vi "Main.vi"() -> ()   [LabVIEW 2019]
uses:
  VIs/Telas.ctl
  VIs/TelaConfig/Configuracao.Variaveis.vi
  Users/Nicole/Downloads/a/ims-desktop/Variaveis/CodOrder.vi
  Users/Nicole/Downloads/a/ims-desktop/Variaveis/WindowAppearance.vi
  Users/Nicole/Downloads/a/ims-desktop/Variaveis/User.vi
panel:
  out "NextScreen":T1
  out "Resize":bool
  out "Code":string
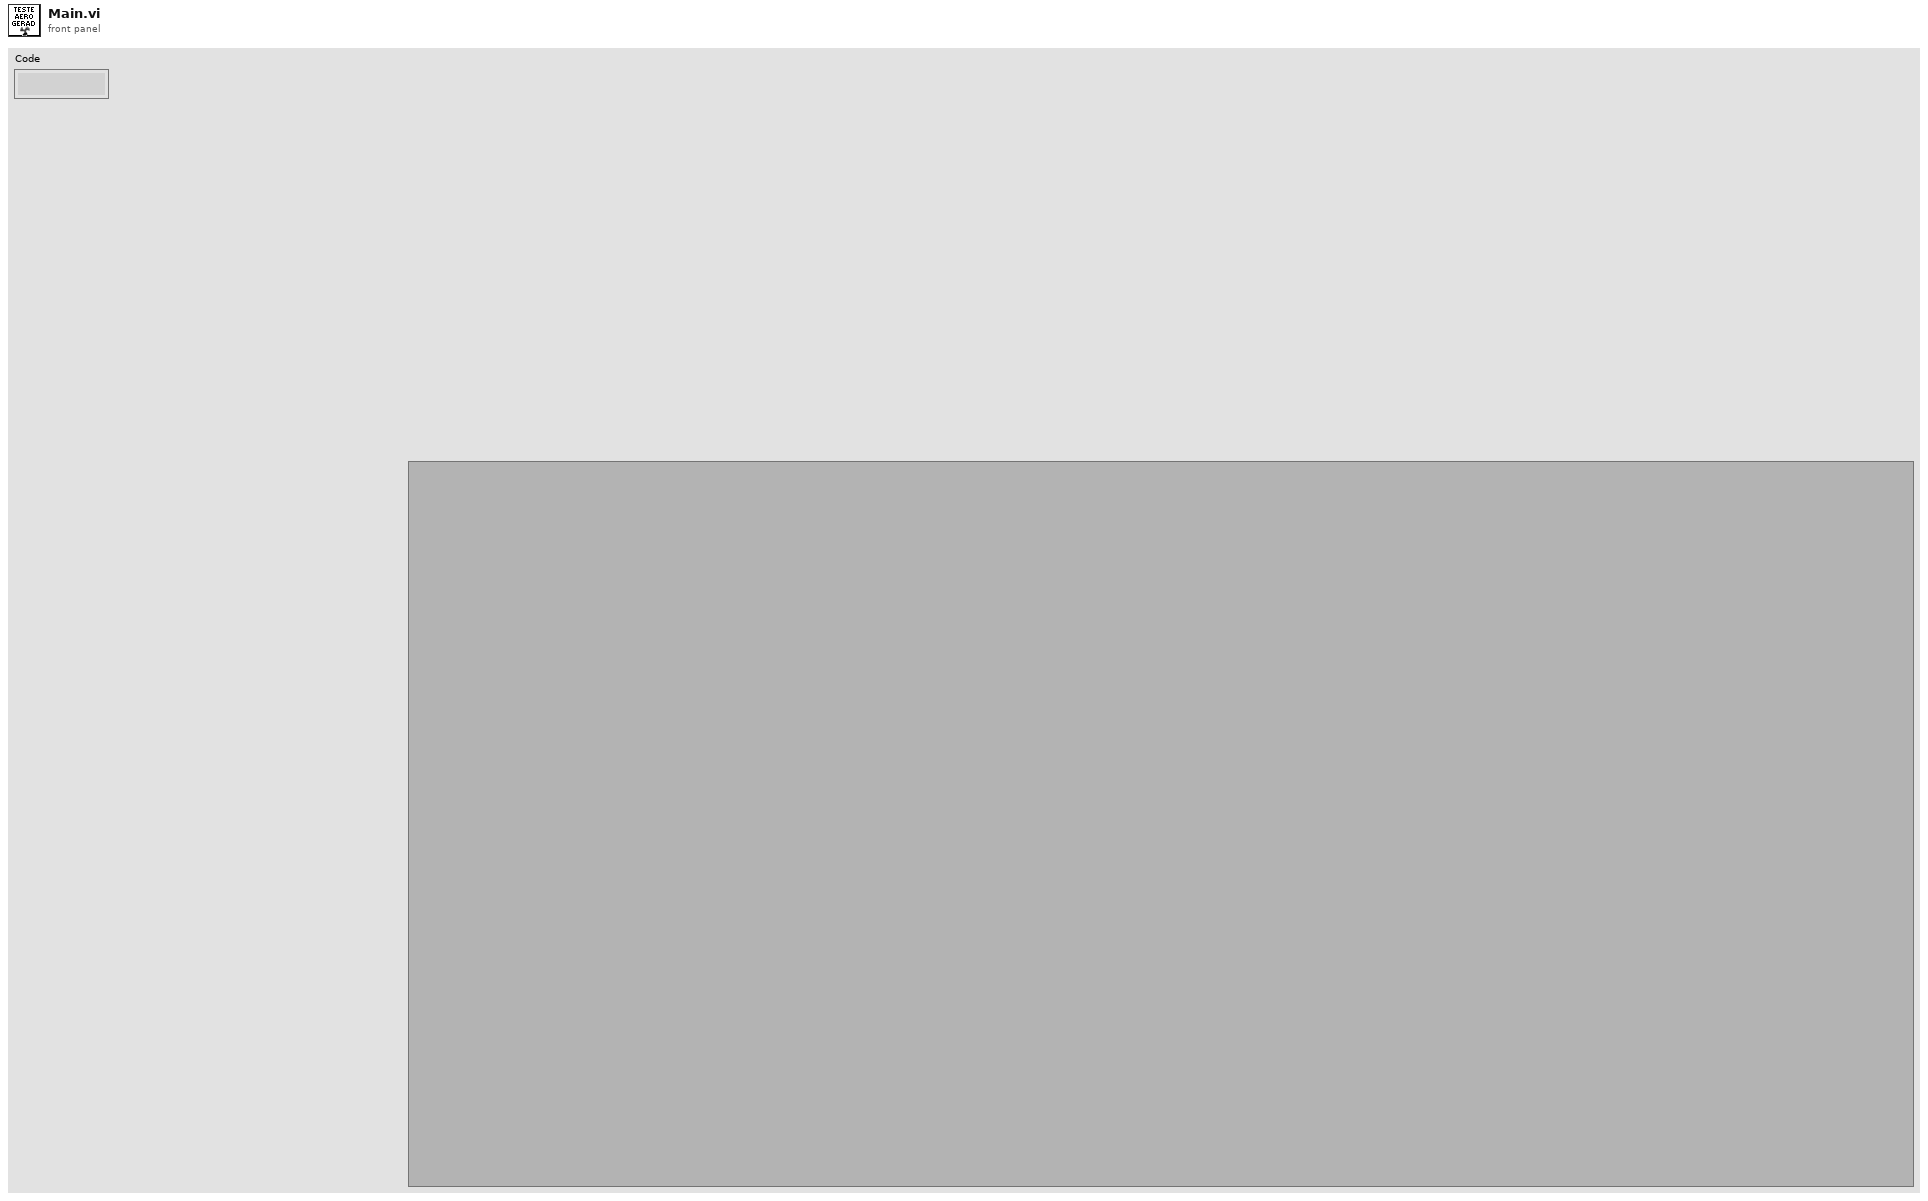
[diagram p1: front panel]
types:
  T1 = typedef "Telas.ctl" = enum16{"Selecao", "Config", "Medicao"}
  T2 = enum32{"invalid app kind", "Development System", "Run Time System", "Student Edition", "Embedded LabVIEW", "Evaluation", "Custom"}
  T3 = typedef "Telas.ctl" = enum16{"Operator", "MeasureFrameTestCommunication", "MeasureFrame", "CNCLoadProgram", "RotorBrokenBars", "Configuration", "MeasureFramePreparation", "WindingLabel", "OtherLabel", "InsulationTapeLabel", "WindingSpecialLabel", "GCF", "AssemblyWindingLabel", "Press", "ThermalProtectorLabel", "Traceability", "MeasureFrameProductionOrder", "MeasureFrameStandardEquipment", "MeasureFrameReferentiate", "LabelScanner", "Alerts", "ProductImages", "QGA", "RotorExternalDiameter", "ComponentRegistration", "WindingInspectionInsulationTapeId", "WindingInspectionPreparation", "WindingInspectionMonitoring", "BearingStiffnessMotorIdentification", "BearingStiffnessLvdtSetup", "BearingStiffness", "WindingInspectionMeasureResistance", "BearingStiffnessManualMode", "Calibration", "PressTooling", "GageDrawing", "BalancingReportProductionOrder", "BalancingReport", "PressMeasureAndControl", "WireFaultDetectionMAG", "StatorImpregnationWeight", "MeasureCapacitance", "SpecialCover", "RegistrationOfInspectionDocuments", "BearingHouseDiameter", "HeaterTemperatureRecord", "PackageLength", "Cnc", "BadgeRegistration", "SpecialFrame", "TerminalBoxFitting", "CoordinateMeasuringMachineDataConversion", "Checklist", "FrameCoverFit", "ShaftGrindingInspection", "ShaftBearingPress", "RotorHeatTreatment", "PressingMeasureBeatPulley", "MotorVisualInspection", "VacuumImpregnation", "Standards", "PaintPreparation", "Runout", "RotorPressingDimension"}
  T4 = enum16{"NoAccess", "Administrator", "Analyst", "Operator"}
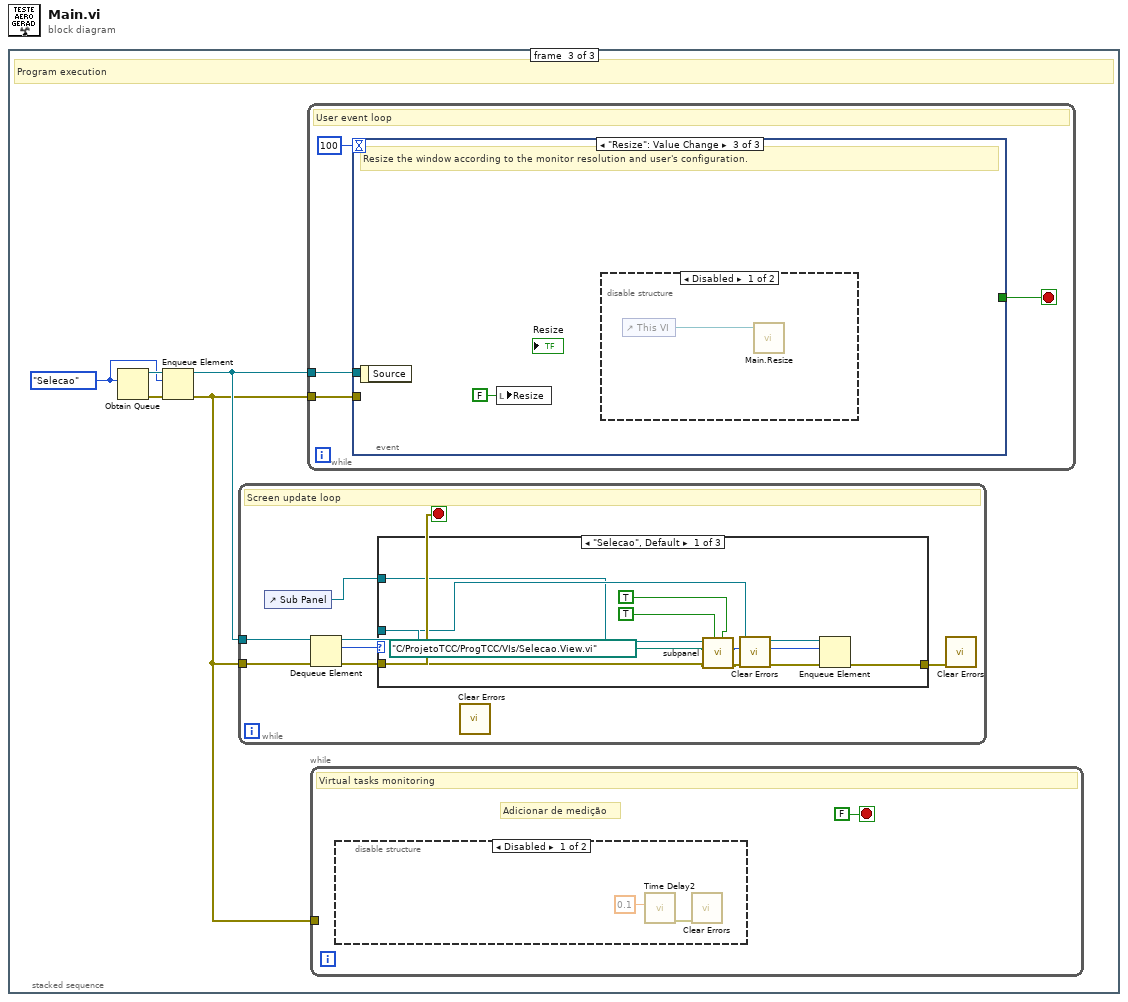
[diagram p0: block diagram]
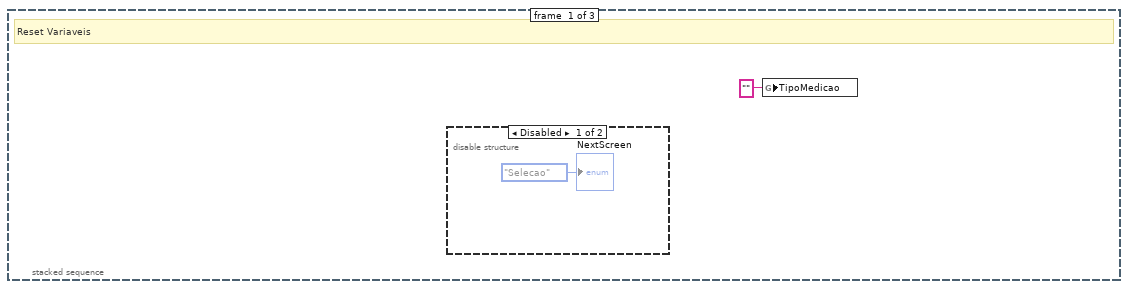
[diagram p2: hidden frame]
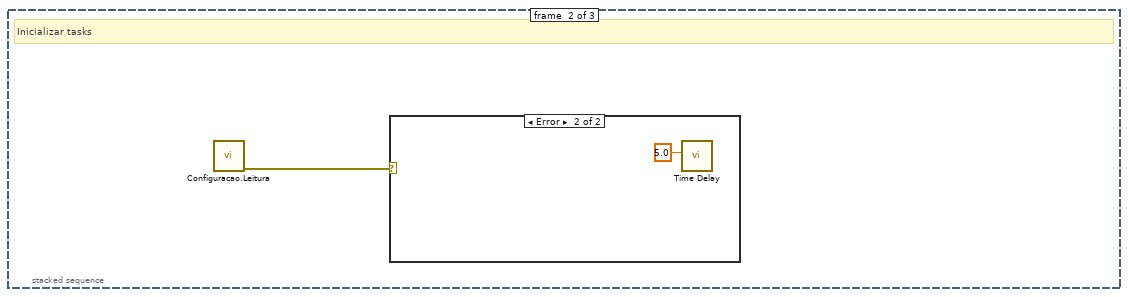
[diagram p4: hidden frame]
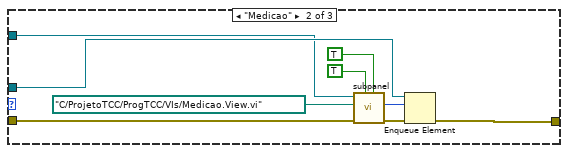
[diagram p7: hidden frame]
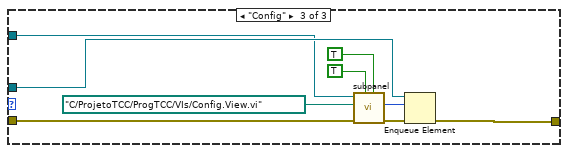
[diagram p8: hidden frame]
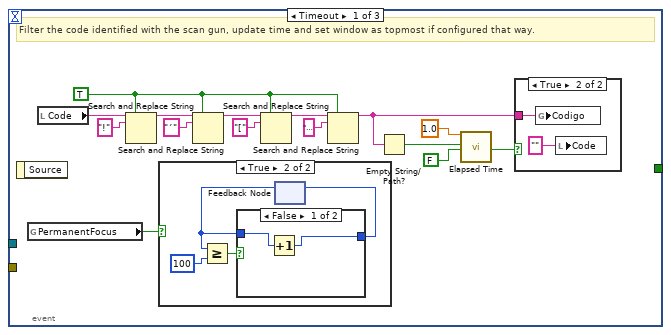
[diagram p9: hidden frame]
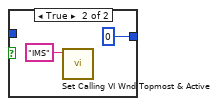
[diagram p11: hidden frame]
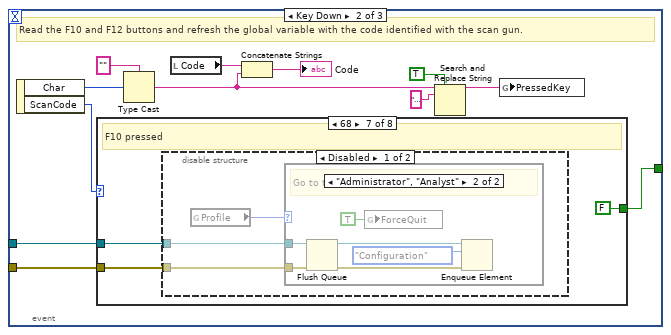
[diagram p13: hidden frame]
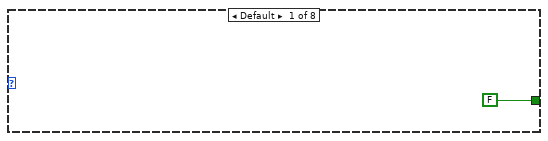
[diagram p14: hidden frame]
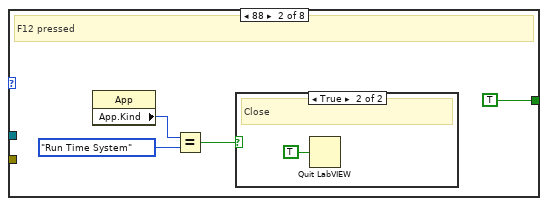
[diagram p15: hidden frame]
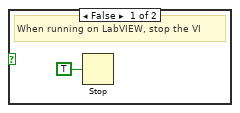
[diagram p16: hidden frame]
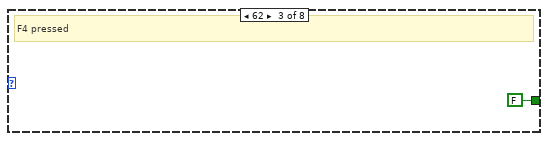
[diagram p17: hidden frame]
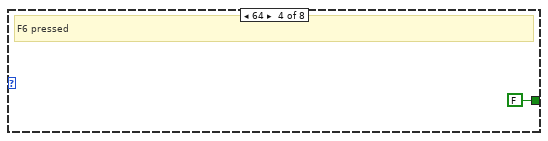
[diagram p18: hidden frame]
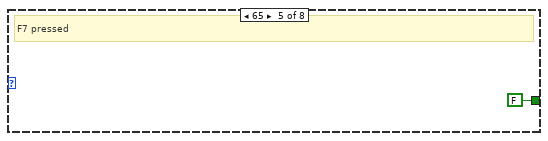
[diagram p19: hidden frame]
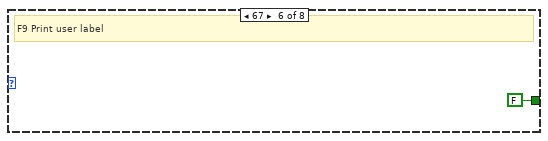
[diagram p20: hidden frame]
diagram:
  n1 = stacked-sequence {
    frame #0 {
      # "Reset Variaveis"
      n2 = disable-structure shown="Disabled" {
        frame Disabled {
          "NextScreen" <- Telas."Selecao" ("NextScreen")
        }
        frame Enabled {
        }
      }
      n3 = global write "Configuracao.Variaveis.vi" "TipoMedicao"("" ("TipoMedicao")) -> ()
    }
    frame #1 {
      # "Inicializar tasks"
      n4 = call "Configuracao.Leitura.vi"() -> ("error out"=w3:errorcluster)  [unwired: 11 in]
      n5 = case shown="Error" w3 {
        frame No Error {
        }
        frame Error {
          n6 = call "Time Delay"("Delay Time (s)"=5.0) -> ()  [unwired: 10 in, 1 out]
        }
      }
    }
    frame #2 {
      w7 = Telas."Selecao" ("NextScreen")
      # "Program execution"
      n7 = Obtain Queue(element data type=w7) -> (queue out=w8:refnum<queue>, error out=w9:errorcluster)  [unwired: 4 in, 1 out]
      n8 = Enqueue Element(queue=w8, element=w7, error in (no error)=w9) -> (queue out=w6:refnum<queue>, error out=w5:errorcluster)  [unwired: 1 in, 1 out]
      n9 = while {
        tunnel: w5 -> [w20]
        tunnel: w6 -> [w19]
        stop <- w18 stop-if-true
        # "Screen update loop"
        n10 = control-ref of="Sub Panel"() -> (w14:refnum<vi>)
        n11 = Dequeue Element(queue=w19, error in (no error)=w20) -> (queue out=w17:refnum<queue>, element=w16:T1, error out=w18:errorcluster)  [unwired: 1 in, 1 out]
        n12 = case shown="\"Selecao\", Default" w16 {
          tunnel: w17 -> [w30 w34 w43]
          tunnel: w18 -> [w23 w33 w42]
          tunnel: w14 -> [w22 w32 w41]
          tunnel: [w29 w31 w40] -> w15
          frame "Selecao", Default {
            n13 = call "subpanel.vi"("Panel Transparent"=TRUE, "Wait Until Done"=TRUE, "error in"=w23, "Vi"=path "C:/ProjetoTCC/ProgTCC/VIs/Selecao.View.vi", "SubPanel"=w22) -> ("error out"=w28:errorcluster, "NextScreen"=w27:T1)  [unwired: 4 in, 1 out]
            n14 = call <vilib>:"Clear Errors.vi"("error in (no error)"=w28) -> ("error out"=w21:errorcluster)  [unwired: 5 in, 1 out]
            n15 = Enqueue Element(queue=w30, element=w27, error in (no error)=w21) -> (error out=w29:errorcluster)  [unwired: 1 in, 2 out]
          }
          frame "Medicao" {
            n16 = call "subpanel.vi"("Panel Transparent"=TRUE, "Wait Until Done"=TRUE, "error in"=w33, "Vi"=path "C:/ProjetoTCC/ProgTCC/VIs/Medicao.View.vi", "SubPanel"=w32) -> ("error out"=w38:errorcluster, "NextScreen"=w39:T1)  [unwired: 4 in, 1 out]
            n17 = Enqueue Element(queue=w34, element=w39, error in (no error)=w38) -> (error out=w31:errorcluster)  [unwired: 1 in, 2 out]
          }
          frame "Config" {
            n18 = call "subpanel.vi"("Panel Transparent"=TRUE, "Wait Until Done"=TRUE, "error in"=w42, "Vi"=path "C:/ProjetoTCC/ProgTCC/VIs/Config.View.vi", "SubPanel"=w41) -> ("error out"=w47:errorcluster, "NextScreen"=w48:T1)  [unwired: 4 in, 1 out]
            n19 = Enqueue Element(queue=w43, element=w48, error in (no error)=w47) -> (error out=w40:errorcluster)  [unwired: 1 in, 2 out]
          }
        }
        n20 = call <vilib>:"Clear Errors.vi"() -> ()  [unwired: 6 in, 2 out]
        n21 = call <vilib>:"Clear Errors.vi"("error in (no error)"=w15) -> ()  [unwired: 5 in, 2 out]
      }
      n22 = while {
        tunnel: w6 -> [w50]
        tunnel: w5 -> [w49]
        stop <- w52 stop-if-true
        # "User event loop"
        n23 = event shown="[2] \"Resize\": Value Change" {
          selector: _ -> [_ _ _]
          dyn-events: _ -> [_ _ _]
          timeout: 100 -> [_ _ _]
          tunnel: [_ w88 _] -> w52
          tunnel: w50 -> [_ w78 _]
          tunnel: w49 -> [_ w79 _]
          event Timeout {
            w56 = TRUE ("replace all? (F)")
            # "Filter the code identified with the scan gun, update time and set window as topmost if configured that way."
            n24 = event-data() -> ()  [unwired: 1 in, 1 out]
            n25 = global read "WindowAppearance.vi" "PermanentFocus"() -> (w53:bool)
            n26 = local read "Code"() -> (w55:string)
            n27 = Search and Replace String(replace all?=w56, input string=w55, search string="!") -> (result string=w59:string)  [unwired: 5 in, 3 out]
            n28 = case shown="True" w53 {
              frame False {
              }
              frame True {
                n29 = feedback #1() -> (w68:i32)  [unwired: 1 in]
                n30 = Greater Or Equal?(x=w68, y=100) -> (x >= y?=w71:bool)
                n31 = case shown="False" w71 {
                  tunnel: [w73 0] -> w69
                  tunnel: w68 -> [w72 _]
                  frame False {
                    n32 = Increment(x=w72) -> (x+1=w73:i32)
                  }
                  frame True {
                    n33 = call "Set Calling VI Wnd Topmost & Active.vi"("WindowName"="IMS") -> ()  [unwired: 10 in, 1 out]
                  }
                }
                n34 = feedback-in #1(w69) -> ()
              }
            }
            n35 = Search and Replace String(replace all?=w56, input string=w59, search string="´") -> (result string=w61:string)  [unwired: 5 in, 3 out]
            n36 = Search and Replace String(replace all?=w56, input string=w61, search string="[") -> (result string=w63:string)  [unwired: 5 in, 3 out]
            n37 = Search and Replace String(replace all?=w56, input string=w63, search string="\u0000") -> (result string=w54:string)  [unwired: 5 in, 3 out]
            n38 = Empty String/Path?(string/path=w54) -> (empty?=w65:bool)
            n39 = call "Elapsed Time"("Time Target (s)"=1.0, "Reset"=w65, "Auto Reset"=FALSE) -> ("Time has Elapsed"=w67:bool)  [unwired: 9 in, 7 out]
            n40 = case shown="True" w67 {
              tunnel: w54 -> [_ w77]
              frame False {
              }
              frame True {
                n41 = global write "CodOrder.vi" "Codigo"(w77) -> ()
                n42 = local write "Code"("") -> ()
              }
            }
          }
          event Key Down {
            # "Read the F10 and F12 buttons and refresh the global variable with the code identified with the scan gun."
            n43 = event-data() -> ("Char"=w87:i16, "ScanCode"=w89:i16)  [unwired: 1 in]
            n44 = case shown="68" w89 {
              tunnel: [FALSE TRUE FALSE FALSE FALSE FALSE FALSE FALSE] -> w88
              tunnel: w79 -> [_ _ _ _ _ _ w102 _]
              tunnel: w78 -> [_ _ _ _ _ _ w101 _]
              frame Default {
              }
              frame 88 {
                # "F12 pressed"
                n45 = property class="App"() -> ("App.Kind"=w93:T2)  [unwired: 2 in, 2 out]
                n46 = Equal?(x=w93, y=T2."Run Time System") -> (x = y?=w91:bool)
                n47 = case shown="True" w91 {
                  frame False {
                    # "When running on LabVIEW, stop the VI"
                    n48 = Stop(stop? (T)=TRUE) -> ()
                  }
                  frame True {
                    # "Close"
                    n49 = Quit LabVIEW(quit? (T)=TRUE) -> ()
                  }
                }
              }
              frame 62 {
                # "F4 pressed"
              }
              frame 64 {
                # "F6 pressed"
              }
              frame 65 {
                # "F7 pressed"
              }
              frame 67 {
                # "F9 Print user label"
              }
              frame 68 {
                # "F10 pressed"
                n50 = disable-structure shown="Disabled" {
                  disable-tunnel: w102 -> [w106 _]
                  disable-tunnel: w101 -> [w105 _]
                  frame Disabled {
                    n51 = global read "User.vi" "Profile"() -> (w104:T4)
                    n52 = case shown="\"Administrator\", \"Analyst\"" w104 {
                      tunnel: w106 -> [_ w112]
                      tunnel: w105 -> [_ w111]
                      frame "NoAccess", Default {
                        # "No access, display an error message."
                        n53 = call "InformationBar.vi"("BlinkAlert"=TRUE, "Message"="Main.NoConfigAccess", "AlertType"=enum16{"Error", "Warning", "Ok", "Time"}."Error") -> ()  [unwired: 8 in, 1 out]
                      }
                      frame "Administrator", "Analyst" {
                        # "Go to the Configuration Screen."
                        n54 = Flush Queue(queue=w111, error in (no error)=w112) -> (queue out=w114:refnum<queue>, error out=w115:errorcluster)  [unwired: 1 out]
                        n55 = global write "CodOrder.vi" "ForceQuit"(TRUE ("ForceQuit")) -> ()
                        n56 = Enqueue Element(queue=w114, element=Telas."Configuration", error in (no error)=w115) -> ()  [unwired: 1 in, 3 out]
                      }
                    }
                  }
                  frame Enabled {
                  }
                }
              }
              frame 87 {
                # "F11 pressed"
              }
            }
            n57 = Type Cast(type="", x=w87) -> (*(type *) &x=w82:string)
            n58 = local read "Code"() -> (w85:string)
            n59 = Concatenate Strings(w85, w82) -> (→"Code":string)
            n60 = Search and Replace String(replace all?=TRUE ("replace all? (F)"), input string=w82, search string="\u0000") -> (result string=w80:string)  [unwired: 5 in, 3 out]
            n61 = global write "CodOrder.vi" "PressedKey"(w80) -> ()
          }
          event "Resize": Value Change {
            # "Resize the window according to the monitor resolution and user's configuration."
            n62 = event-data() -> ()  [unwired: 1 in, 1 out]
            n63 = local write "Resize"(FALSE ("Resize")) -> ()
            n64 = disable-structure shown="Disabled" {
              frame Disabled {
                n65 = control-ref of="This VI"() -> (w119:refnum<vi>)
                n66 = call "Main.Resize.vi"("VI in"=w119) -> ("Sub Panel"=w118:refnum<vi>)  [unwired: 10 in]
              }
              frame Enabled {
              }
            }
          }
        }
      }
      n67 = while {
        tunnel: w5 -> [_]
        stop <- FALSE stop-if-true
        # "Adicionar de medição"
        # "Virtual tasks monitoring"
        n68 = disable-structure shown="Disabled" {
          frame Disabled {
            n69 = call "Time Delay2"("Delay Time (s)"=0.1) -> ("error out"=w11:errorcluster, "error in (no error)"=w12:errorcluster)  [unwired: 9 in]
            n70 = call <vilib>:"Clear Errors.vi"("error in (no error)"=w11) -> ()  [unwired: 5 in, 2 out]
          }
          frame Enabled {
          }
        }
      }
    }
  }
